vi "1D Fit Simulate Data.vi"(8 "Error In":errorcluster, 9 "Model Parameters":variant, 11 "Simulation Options":T2) -> (0 "Error Out":errorcluster, 3 "Plot":T1)   [LabVIEW 2021, in "Fits.lvlib"]
uses:
  1D Fit Simulation Options.ctl
  Fit Models.ctl
  Graphs/XY Graph/XY Plot Data.ctl
  07a11e08-f6d2-4209-80e3-4982b1dcfee3.vi
  2da1e5ea-9d91-461e-a147-628295f3f3b8.vi
  2da1e5ea-9d91-461e-a147-628295f3f3b8.vi/539bd7ec-d9e8-460f-a56d-a449b4a86a5e.vi
  <vilib>/gmath/statdist.llb/Normal Random.vi
  <vilib>/gmath/statdist.llb/Poisson Random.vi
  Fits.lvlib
  <vilib>/gmath/NI_Gmath.lvlib
  Error/Error.lvlib
  Graphs/XY Graph/XY Graph Add-Ons.lvlib
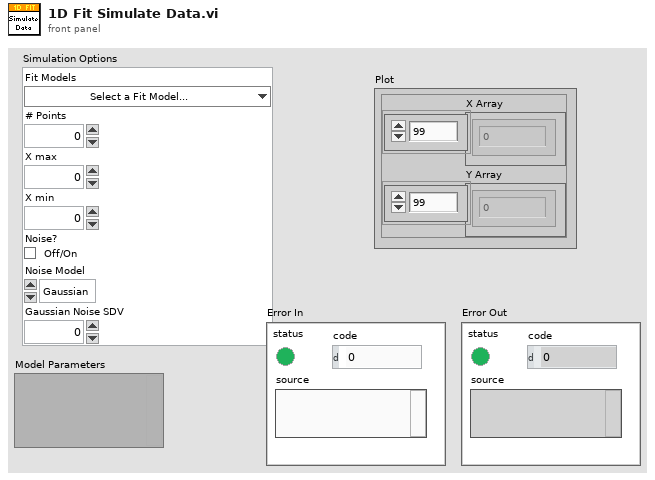
[diagram p1: front panel]
types:
  T1 = typedef "XY Graph Add-Ons.lvlib/XY Plot Data.ctl" = cluster{"X Array":dbl[], "Y Array":dbl[]}
  T2 = typedef "Fits.lvlib/1D Fit Simulation Options.ctl" = cluster{"Fit Models":T3, "# Points":i32, "X max":dbl, "X min":dbl, "Noise?":bool, "Noise Model":enum16{"Gaussian", "Poisson"}, "Gaussian Noise SDV":dbl}
  T3 = typedef "Fits.lvlib/Fit Models.ctl" = enum16{"Select a Fit Model...", "           Single Peak", "Gaussian", "Asymmetric Gaussian", "Lorentzian", "Asymmetric Lorentzian", "Gaussian/Lorentzian", "Lorentzian/Gaussian", "           Double Peak", "Two Gaussians", "Two Asymmetric Gaussians", "Two H-Connected Gaussians", "Two T-Connected Gaussians", "Two H-Connected Asymmetric Gaussians", "Two T-Connected Asymmetric Gaussians", "           Triple Peak", "Three Gaussians", "Three Asymmetric Gaussians", "              Decays", "1-Exponential", "IRF*PSED", "2-Exponentials", "Power Law", "               ACF", "2D Gaussian ACF", "2D Gaussian + Blinking ACF", "2D Gaussian + Flow ACF", "3D Gaussian ACF", "3D Gaussian + Blinking ACF", "             Multiplot", "2D Gaussian ACF & 2D Gaussian + Flow ACF"}
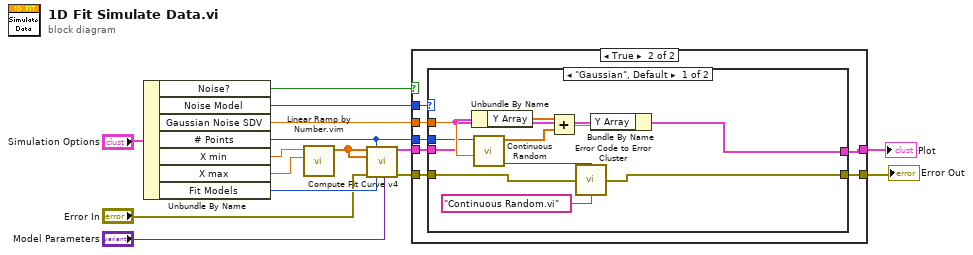
[diagram p0: block diagram]
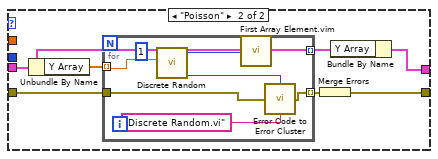
[diagram p3: hidden frame]
diagram:
  n1 = Unbundle By Name("Simulation Options") -> ("Noise?"=w8:bool, "Noise Model"=w5:enum16{"Gaussian", "Poisson"}, "Gaussian Noise SDV"=w4:dbl, "# Points"=w3:i32, "X min"=w14:dbl, "X max"=w13:dbl, "Fit Models"=w11:T3)
  n2 = call "Linear Ramp by Number.vim"("End (1)"=w13, "Start (0)"=w14) -> ("Ramp"=w9:dbl[])  [unwired: 7 in, 2 out]
  n3 = call "Compute Fit Curve v4.vi"("X Array in"=w9, "# Points"=w3, "Best Fit in"=w9, "Error In"="Error In", "Fit Model"=w11, "Fit Parameters"="Model Parameters") -> ("Fitted Plot"=w7:cluster{"X Array":dbl[], "Y Array":dbl[]}, "Error Out"=w2:errorcluster)  [unwired: 4 in, 4 out]
  n4 = case shown="True" w8 {
    tunnel: w7 -> [w17 w20]
    tunnel: [w17 w19] -> w6
    tunnel: w5 -> [_ w24]
    tunnel: w4 -> [_ w23]
    tunnel: w3 -> [_ w22]
    tunnel: w2 -> [w16 w21]
    tunnel: [w16 w18] -> w1
    frame False {
    }
    frame True {
      n5 = case shown="\"Gaussian\", Default" w24 {
        tunnel: w23 -> [w35 _]
        tunnel: w22 -> [w34 _]
        tunnel: w21 -> [w28 w41]
        tunnel: w20 -> [w33 w38]
        tunnel: [w32 w36] -> w19
        tunnel: [w26 w39] -> w18
        frame "Gaussian", Default {
          n6 = Unbundle By Name(w33) -> ("Y Array"=w31:dbl[])
          n7 = call-poly <vilib>:"Continuous Random.vi"("std"=w35, "samples"=w34) -> ("error"=w27:i32, "normal random data"=w30:dbl[])  [unwired: 8 in]
          n8 = Add(x=w31, y=w30) -> (x+y=w29:dbl[])
          n9 = call "Error Code to Error Cluster.vi"("Error Code"=w27, "Error Source"="Continuous Random.vi", "Error In"=w28) -> ("Error Out"=w26:errorcluster)  [unwired: 12 in]
          n10 = Bundle By Name(cluster=w33, "Y Array"=w29) -> (w32:cluster{"X Array":dbl[], "Y Array":dbl[]})
        }
        frame "Poisson" {
          n11 = Unbundle By Name(w38) -> ("Y Array"=w42:dbl[])
          n12 = for {
            tunnel: w42 -> [w49] mode=indexing
            tunnel: w41 -> [w47]
            tunnel: [w46] -> w40 mode=indexing
            tunnel: [w43] -> w37 mode=indexing
            n13 = call-poly <vilib>:"Discrete Random.vi"("lambda"=w49, "samples"=1) -> ("error"=w48:i32, "Poisson random data"=w44:i32[])  [unwired: 8 in]
            n14 = call "First Array Element.vim"("Array"=w44) -> ("First Element"=w43:i32)  [unwired: 8 in]
            n15 = call "Error Code to Error Cluster.vi"("Error Code"=w48, "Error Source"="Discrete Random.vi", "Error In"=w47) -> ("Error Out"=w46:errorcluster)  [unwired: 12 in]
          }
          n16 = Merge Errors(w40) -> (w39:errorcluster)
          n17 = Bundle By Name(cluster=w38, "Y Array"=w37) -> (w36:cluster{"X Array":dbl[], "Y Array":dbl[]})
        }
      }
    }
  }
  "Error Out" <- w1
  "Plot" <- w6
